vi "Threshold-Image to Binary.vi"(8 "error in (no error)":errorcluster, 11 "Image source":T1) -> (0 "Error out at image plane extraction and threshold":errorcluster, 3 "Binary Image after threshold":T1(plugin-control))   [LabVIEW 2016]
uses:
  <vilib>/vision/Image Controls.llb/IMAQ Image.ctl
  <vilib>/vision/NI_Vision_Development_Module.lvlib
panel:
  in  "Keep/Replace Value (Replace)":bool=TRUE
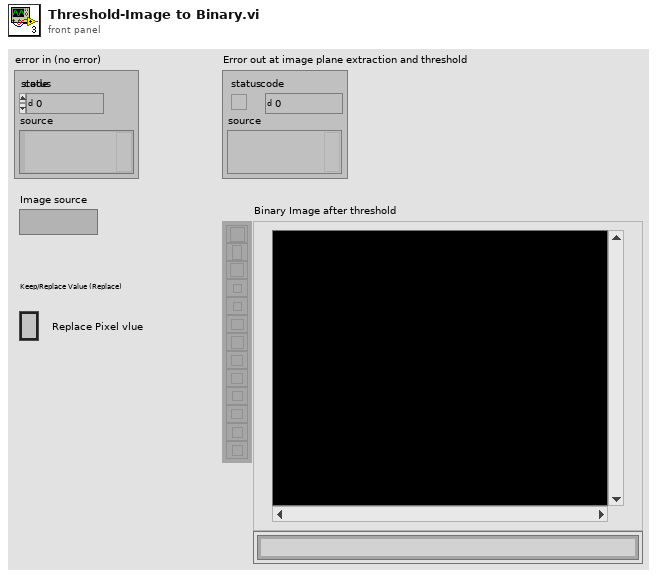
[diagram p1: front panel]
types:
  T1 = typedef "IMAQ Image.ctl" = refnum<image>
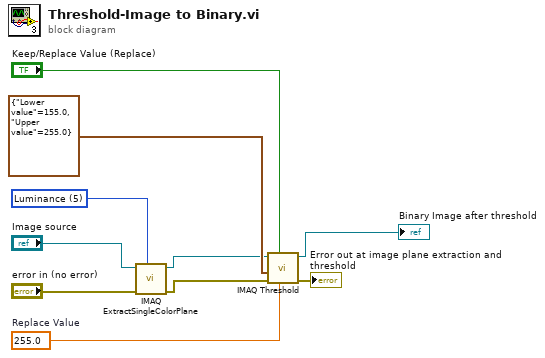
[diagram p0: block diagram]
diagram:
  w5 = sgl 255.0  # Replace Value
  w8 = 5 items=["Red", "Green", "Blue", "Hue", "Saturation", "Luminance", "Value", "Intensity"] ("Color Plane")
  n1 = call "IMAQ ExtractSingleColorPlane"("Color Plane"=w8, "error in (no error)"="error in (no error)", "Image Src"="Image source") -> ("error out"=w7:errorcluster, "Image Dst Out"=w4:T1)  [unwired: 7 in]
  n2 = call "IMAQ Threshold"("Replace Value"=w5, "Keep/Replace Value (Replace)"="Keep/Replace Value (Replace)", "error in (no error)"=w7, "Range"=cluster{"Lower value":sgl, "Upper value":sgl} {"Lower value"=155.0, "Upper value"=255.0}, "Image Src"=w4) -> ("error out"=→"Error out at image plane extraction and threshold":errorcluster, "Image Dst Out"=→"Binary Image after threshold":T1)  [unwired: 5 in]
